vi "Panel.vi"(11 "VerticalSliderControlEditorPanel in":refnum<class "VerticalSliderControlEditorPanel.lvclass">) -> ()   [LabVIEW 2020, in "VolatusGUIControls.lvlib" / "VerticalSliderControlEditorPanel.lvclass"]
uses:
  VerticalSliderControlEditorPanel.lvclass
  C:/dev/lv20CE/relink/volatus-gui-controls/VolatusGUIEditorCore/ElementEditorPanel/ElementEditorPanel.lvclass
  C:/dev/lv20CE/relink/lv-oopanel/OOPanel/Panel/Panel.lvclass
  VolatusGUIEditorCore/Fill Style.ctl
  lv-oopanel/OOPanel/Panel/Basic UI State.ctl
  lv-autocomplete/AutoComplete/AutoComplete/AutoComplete.lvclass/AutoComplete.ctl
  VerticalSliderControlEditorPanel.lvclass/VerticalSliderControlEditorPanel.ctl
  VolatusGUIEditorCore/Slider Props.ctl
  lv-autocomplete/AutoComplete/Launch Autocomplete Handler.vi
  lv-autocomplete/AutoComplete/AutoComplete/AutoComplete.lvclass
  lv-oopanel/OOPanel/Panel/Panel.lvclass
  lv-oopanel/OOPanel/OOPanel.lvlib
  VolatusGUIEditorCore/ElementEditorPanel/ElementEditorPanel.lvclass
  VolatusGUIEditorCore/VolatusGUIEditorCore.lvlib
panel:
  in  "Inhibit":string caption="Channel"
  in  "Max":dbl
  in  "Min":dbl
  in  "Slider Color":u32(colorbox) caption="Slider"
  in  "Fill":T1
  in  "Height":u16
  in  "BG Color":u32(colorbox) caption="BG"
  in  "Fill Color":u32(colorbox) caption="Fill"
  in  "Top":i32
  in  "Left":i32
  in  "Width":u16
  in  "Label Text Color":u32(colorbox) caption="Color"
  in  "Label Visible":bool caption="Visible"
  in  "Label":string
  in  "Channel":string
  # "Label"
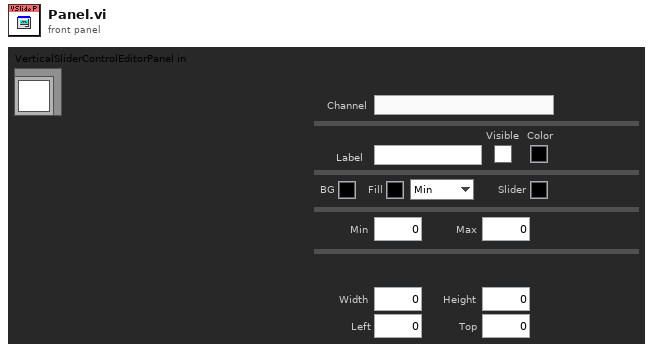
[diagram p1: front panel]
types:
  T1 = typedef "VolatusGUIEditorCore.lvlib/Fill Style.ctl" = enum16{"Min", "Max", "None"}
  T2 = typedef "OOPanel.lvlib/Panel.lvclass/Basic UI State.ctl" = enum16{"Init", "Run", "Close"}
  T3 = typedef "VolatusGUIEditorCore.lvlib/Slider Props.ctl" = cluster{"Fill Color":u32, "BG Color":u32, "Slider Color":u32, "Fill Style":T1, "Min":dbl, "Max":dbl}
  T4 = typedef "VolatusGUIEditorCore.lvlib/ElementEditorPanel.lvclass/Incoming Events.ctl" = cluster{"Update Control":refnum<user-event>}
  T5 = typedef "OOPanel.lvlib/Panel.lvclass/Panel Events.ctl" = cluster{"Visbility":refnum<user-event>, "Close":refnum<user-event>}
  T6 = typedef "VolatusGUIControls.lvlib/VerticalSliderControlEditorPanel.lvclass/Props.ctl" = cluster{"JSON":T7, "Label":T8, "Position":T9, "Width":u16, "Height":u16, "Slider":T3}
  T7 = typedef "VolatusGUIControls.lvlib/VerticalSliderControlEditorPanel.lvclass/JSON Props.ctl" = cluster{"Channel":string, "Inhibit":string}
  T8 = typedef "VolatusGUIEditorCore.lvlib/Label Props.ctl" = cluster{"Text":string, "Text Color":u32, "Visible":bool}
  T9 = typedef "VolatusGUIEditorCore.lvlib/Position Props.ctl" = cluster{"Left":i32, "Top":i32}
  T10 = typedef "OOPanel.lvlib/Visibility State.ctl" = enum16{"Idle", "Closed", "Hidden", "Visible", "Subpanel", "Hidden Subpanel"}
  T11 = cluster{"Label":string, "Label Text Color":u32, "Label Visible":bool}
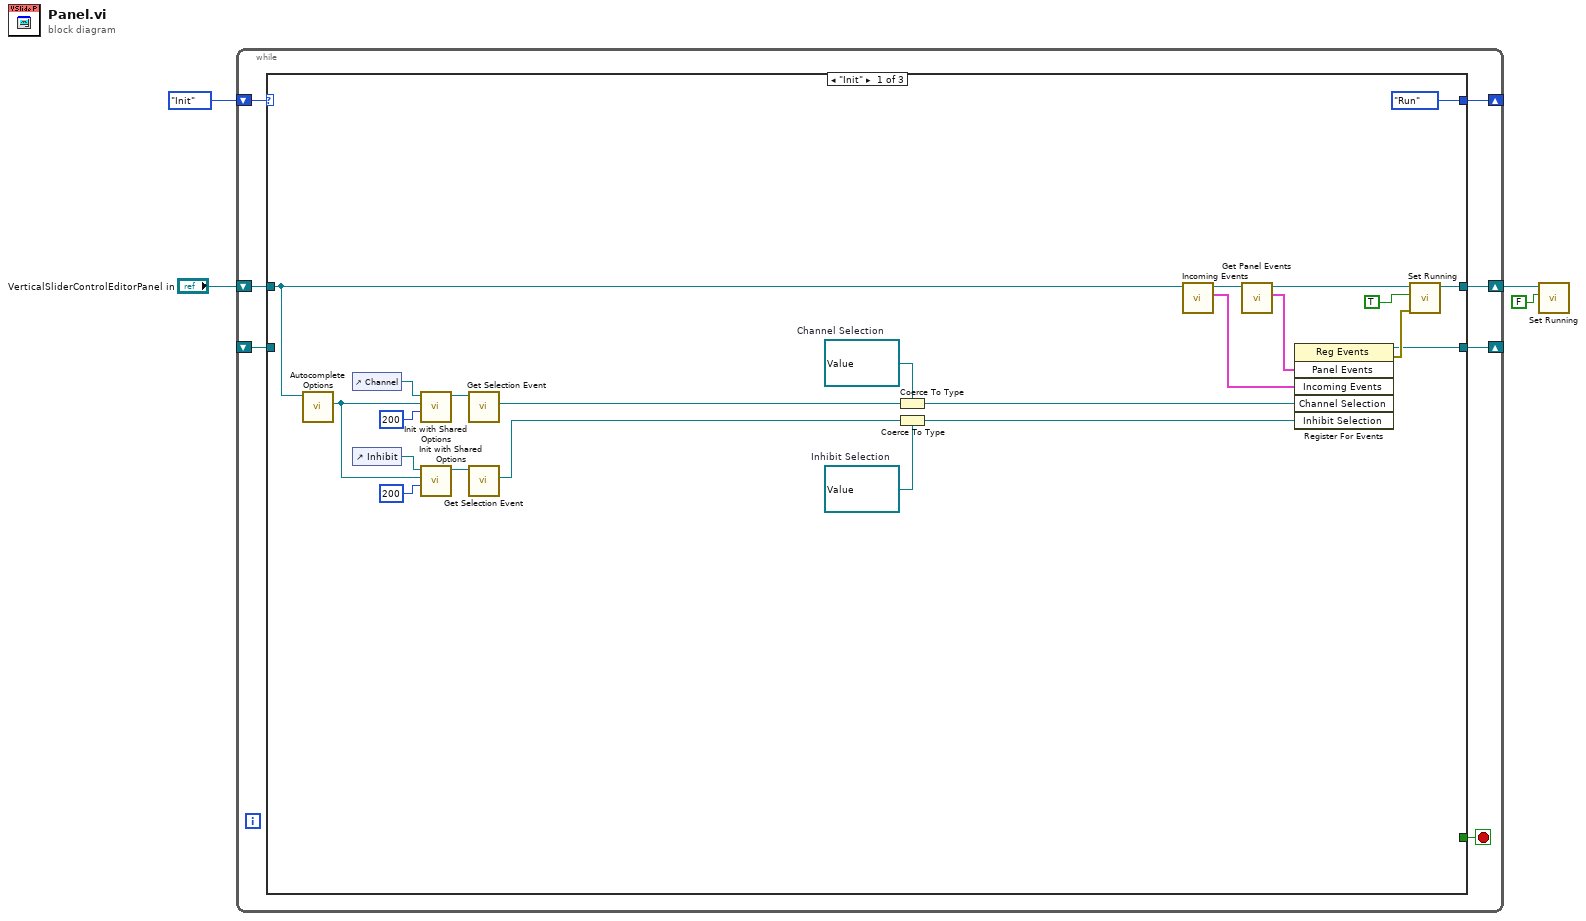
[diagram p0: block diagram]
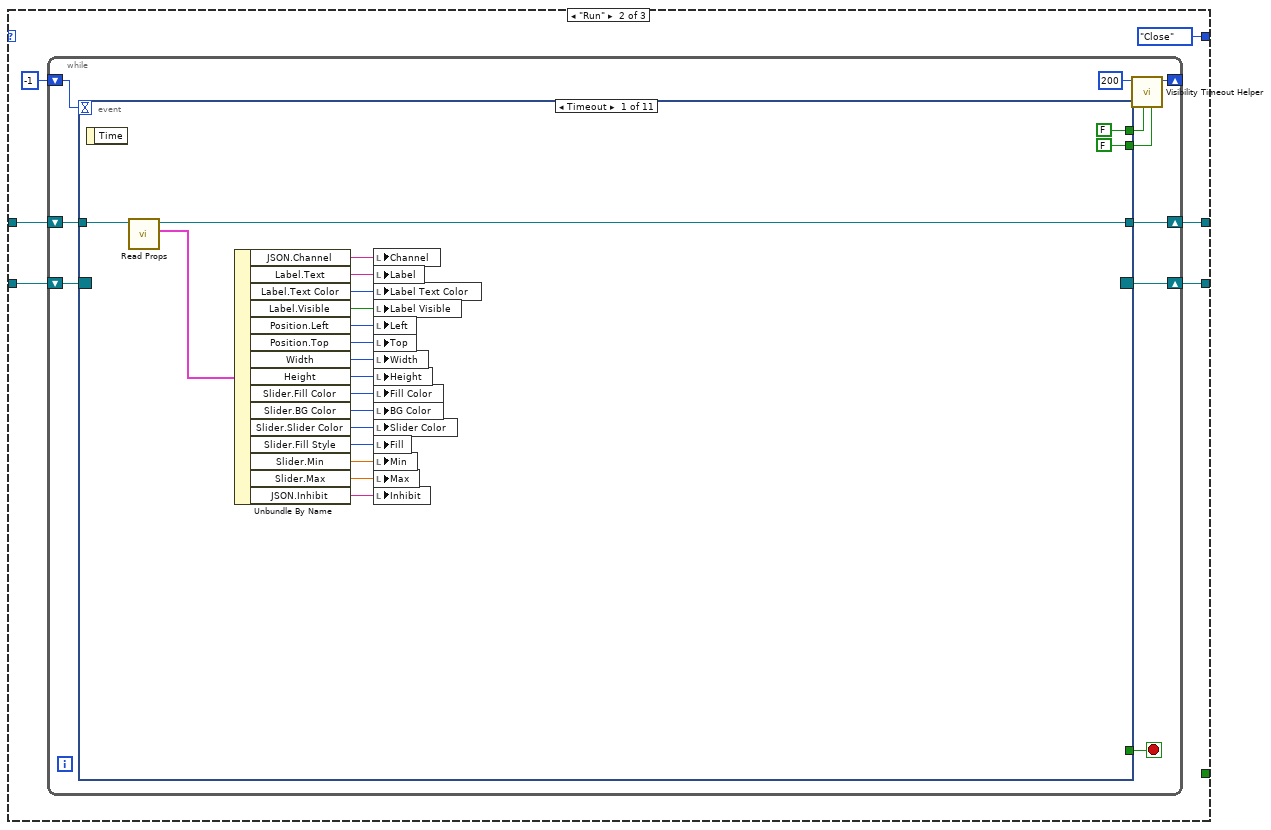
[diagram p2: hidden frame]
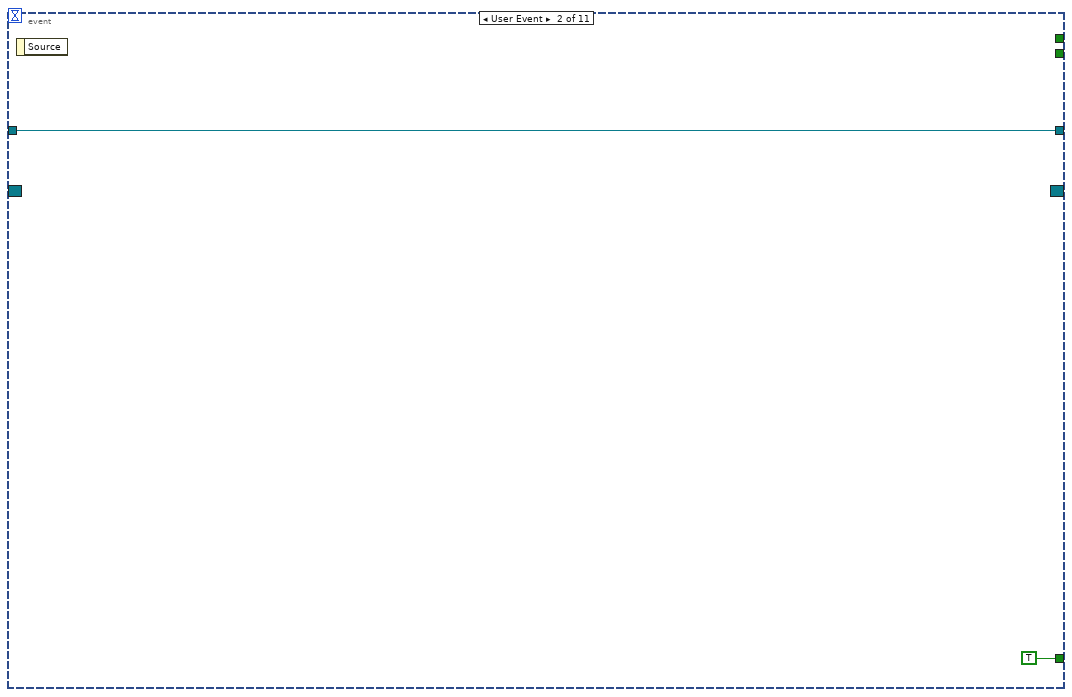
[diagram p3: hidden frame]
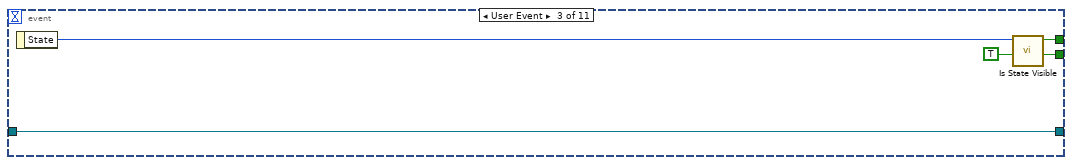
[diagram p4: hidden frame]
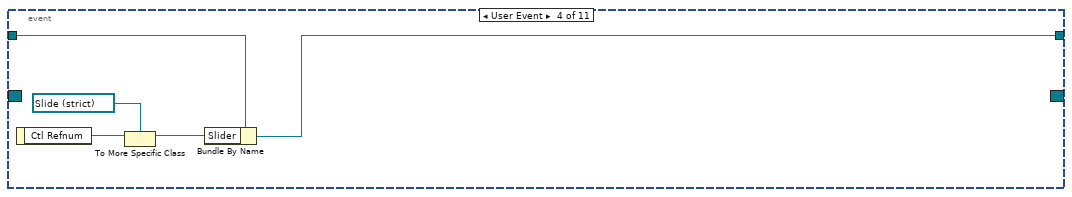
[diagram p5: hidden frame]
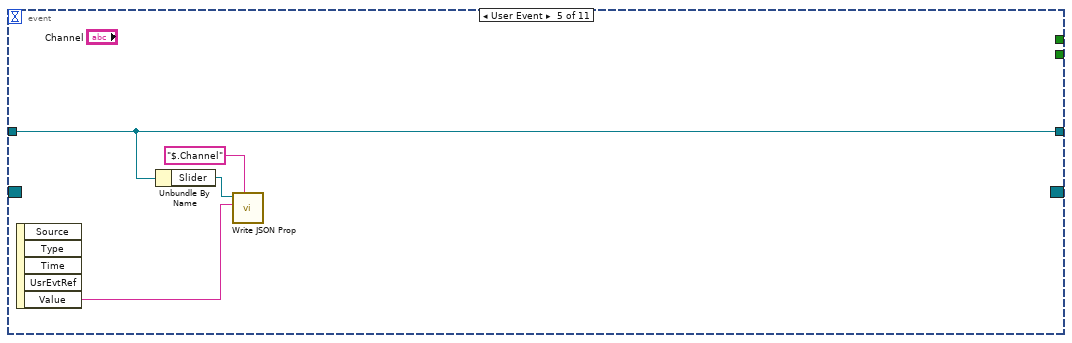
[diagram p6: hidden frame]
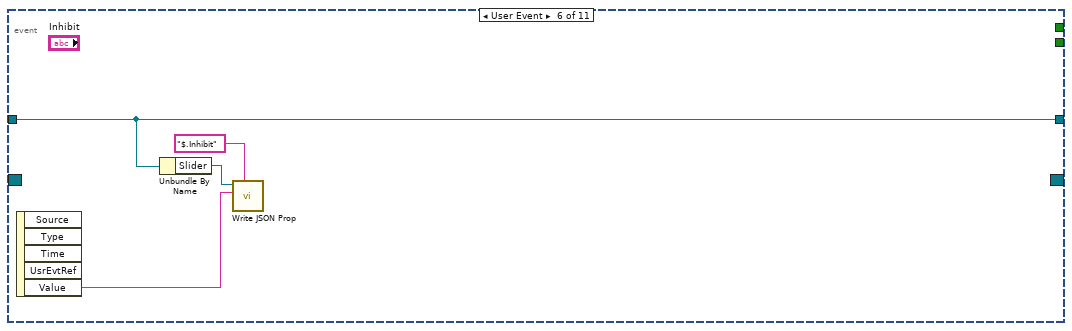
[diagram p7: hidden frame]
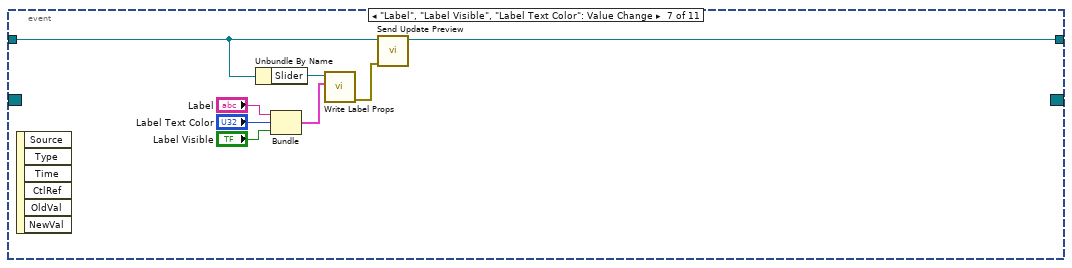
[diagram p8: hidden frame]
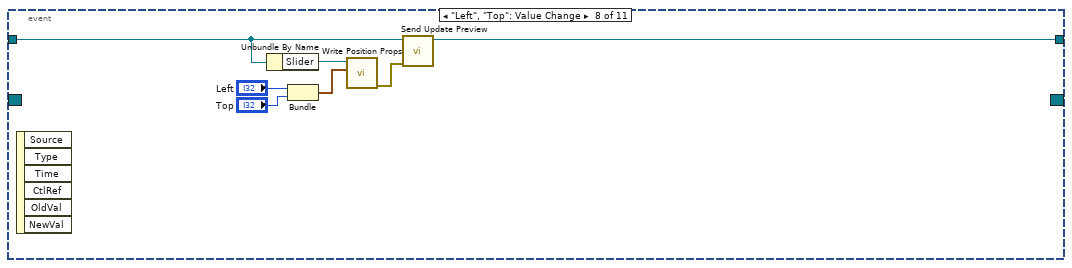
[diagram p9: hidden frame]
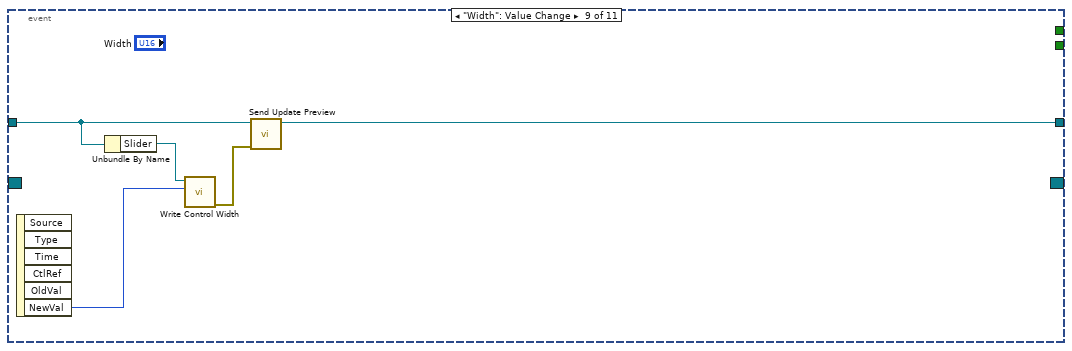
[diagram p10: hidden frame]
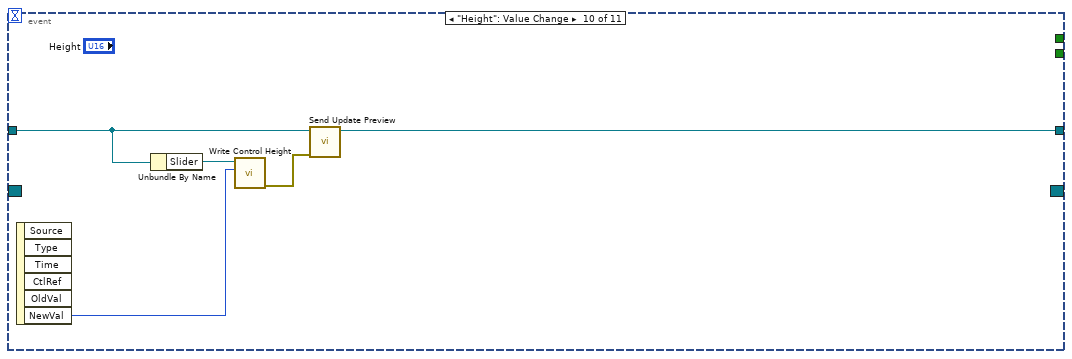
[diagram p11: hidden frame]
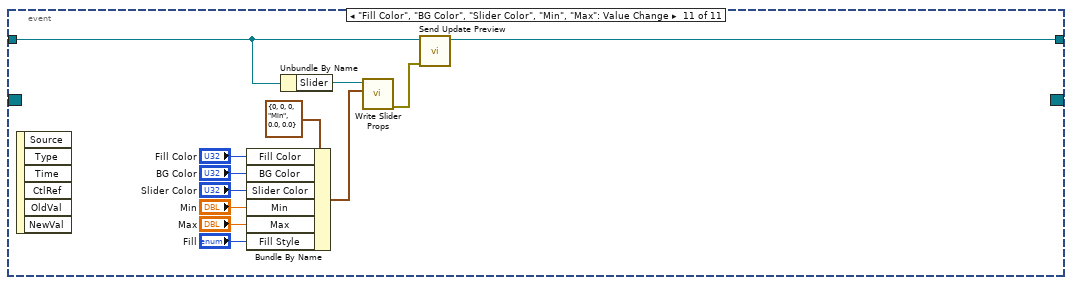
[diagram p12: hidden frame]
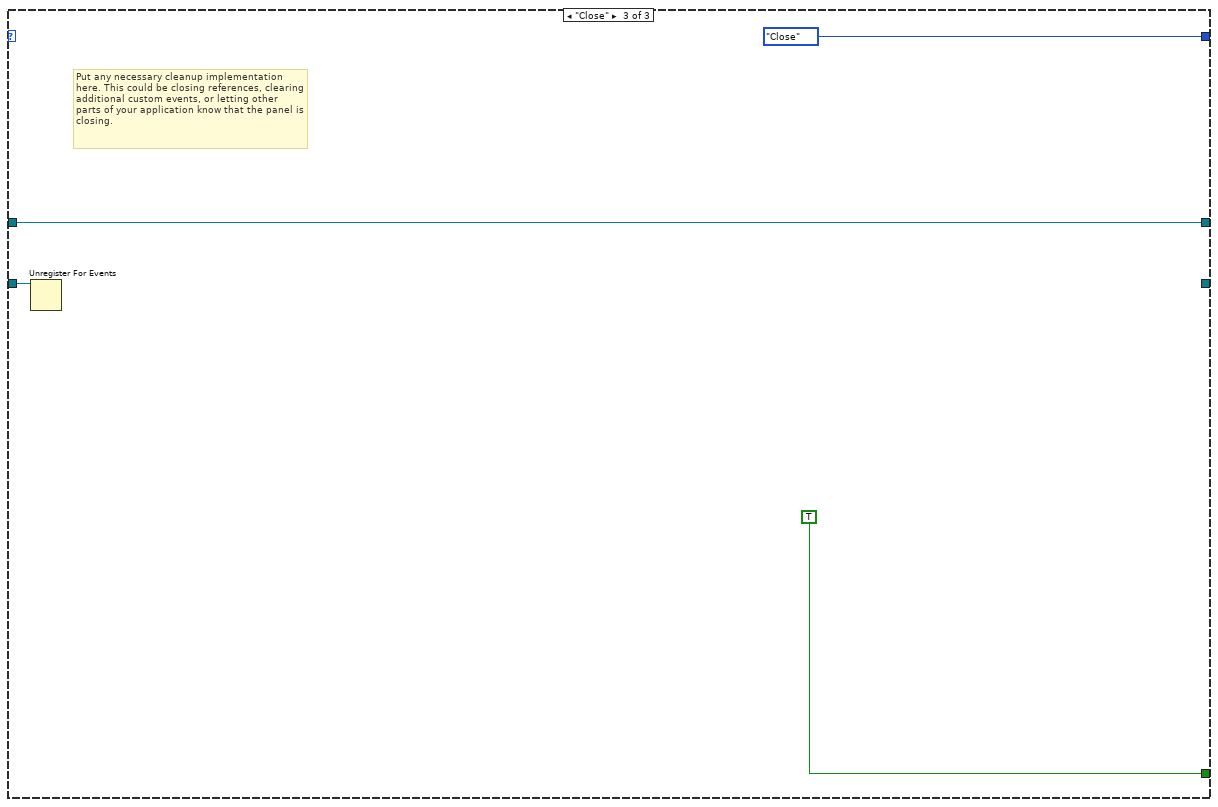
[diagram p13: hidden frame]
diagram:
  n1 = while {
    shift-right: [w10] -> _
    shift-left: _ -> [w11]
    shift-right: [w8] -> _
    shift-left: Basic_UI_State."Init" ("Basic UI State") -> [w9]
    shift-right: [w6] -> w4
    shift-left: "VerticalSliderControlEditorPanel in" -> [w5]
    stop <- w7 stop-if-true
    n2 = case shown="\"Init\"" w9 {
      tunnel: w11 -> [_ w40 w128]
      tunnel: [w31 w38 _] -> w10
      tunnel: [Basic_UI_State."Run" ("Basic UI State") Basic_UI_State."Close" ("Basic UI State") Basic_UI_State."Close" ("Basic UI State")] -> w8
      tunnel: [_ _ TRUE] -> w7
      tunnel: [w30 w35 w127] -> w6
      tunnel: w5 -> [w23 w36 w127]
      frame "Init" {
        w13 = refnum<user-event> refnum  # Inhibit Selection
        w15 = refnum<user-event> refnum  # Channel Selection
        n3 = call "Autocomplete Options.vi"("ElementEditorPanel in"=w23) -> ("Autocomplete Options"=w19:refnum<class "Shared Options.lvclass">)  [unwired: 10 in]
        n4 = control-ref of="Channel"() -> (w22:refnum<vi>)
        n5 = control-ref of="Inhibit"() -> (w17:refnum<vi>)
        n6 = call "Init with Shared Options.vi"("Height (200)"=i16 200, "Shared Options"=w19, "Str Refnum"=w22) -> ("AutoComplete out"=w24:refnum<class "AutoComplete.lvclass">)  [unwired: 7 in, 1 out]
        n7 = call "Init with Shared Options.vi"("Height (200)"=i16 200, "Shared Options"=w19, "Str Refnum"=w17) -> ("AutoComplete out"=w18:refnum<class "AutoComplete.lvclass">)  [unwired: 7 in, 1 out]
        n8 = call "Get Selection Event.vi"("AutoComplete in"=w24) -> ("Selection Event"=w21:refnum<user-event>)  [unwired: 9 in, 1 out]
        n9 = call "Get Selection Event.vi"("AutoComplete in"=w18) -> ("Selection Event"=w12:refnum<user-event>)  [unwired: 9 in, 1 out]
        n10 = Coerce To Type(0:w21, 1:w15) -> (2:w16:refnum<user-event>)
        n11 = Coerce To Type(0:w12, 1:w13) -> (2:w14:refnum<user-event>)
        n12 = call "Incoming Events.vi"("ElementEditorPanel in"=w23) -> ("Incoming Events"=w26:T4, "ElementEditorPanel out"=w27:refnum<class "VerticalSliderControlEditorPanel.lvclass">)  [unwired: 9 in]
        n13 = call "Get Panel Events.vi"("Panel in"=w27) -> ("Panel Events"=w28:T5, "Panel out"=w29:refnum<class "VerticalSliderControlEditorPanel.lvclass">)  [unwired: 8 in, 1 out]
        n14 = register-events(w28, w26, w16, w14) -> (reference out=w31:refnum<event-registration>, error out=w33:errorcluster)  [unwired: 2 in]
        n15 = call "Set Running.vi"("error in (no error)"=w33, "Running"=TRUE, "Panel in"=w29) -> ("Panel out"=w30:refnum<class "VerticalSliderControlEditorPanel.lvclass">)  [unwired: 7 in, 1 out]
      }
      frame "Run" {
        n16 = while {
          shift-right: [w46] -> w38
          shift-left: w40 -> [w47]
          shift-right: [w49] -> _
          shift-left: -1 ("Timeout") -> [w48]
          shift-right: [w41] -> w35
          shift-left: w36 -> [w42]
          stop <- w43 stop-if-true
          n17 = event shown="[0] Timeout" {
            selector: w47 -> [_ _ _ _ _ _ _ _ _ _ _]
            dyn-events: [_ _ _ _ _ _ _ _ _ _ _] -> w46
            timeout: w48 -> [_ _ _ _ _ _ _ _ _ _ _]
            tunnel: [FALSE _ w75 _ _ _ _ _ _ _ _] -> w45
            tunnel: [FALSE _ TRUE _ _ _ _ _ _ _ _] -> w44
            tunnel: [_ TRUE _ _ _ _ _ _ _ _ _] -> w43
            tunnel: w42 -> [w67 w71 w73 w81 w83 w87 w97 w102 w109 w114 w119]
            tunnel: [w68 w71 w73 w78 w83 w87 w91 w99 w106 w111 w116] -> w41
            event Timeout {
              n18 = event-data() -> ()  [unwired: 1 in, 1 out]
              n19 = call "Read Props.vi"("VerticalSliderControlEditorPanel in"=w67) -> ("Props"=w66:T6, "VerticalSliderControlEditorPanel out"=w68:refnum<class "VerticalSliderControlEditorPanel.lvclass">)  [unwired: 8 in, 1 out]
              n20 = Unbundle By Name(w66) -> ("JSON.Channel"=w65:string, "Label.Text"=w63:string, "Label.Text Color"=w62:u32, "Label.Visible"=w61:bool, "Position.Left"=w60:i32, "Position.Top"=w59:i32, "Width"=w58:u16, "Height"=w57:u16, "Slider.Fill Color"=w56:u32, "Slider.BG Color"=w55:u32, "Slider.Slider Color"=w54:u32, "Slider.Fill Style"=w53:T1, "Slider.Min"=w52:dbl, "Slider.Max"=w64:dbl, "JSON.Inhibit"=w51:string)
              n21 = local write "Channel"(w65) -> ()
              n22 = local write "Label"(w63) -> ()
              n23 = local write "Label Text Color"(w62) -> ()
              n24 = local write "Label Visible"(w61) -> ()
              n25 = local write "Left"(w60) -> ()
              n26 = local write "Top"(w59) -> ()
              n27 = local write "Width"(w58) -> ()
              n28 = local write "Height"(w57) -> ()
              n29 = local write "Fill Color"(w56) -> ()
              n30 = local write "BG Color"(w55) -> ()
              n31 = local write "Slider Color"(w54) -> ()
              n32 = local write "Fill"(w53) -> ()
              n33 = local write "Min"(w52) -> ()
              n34 = local write "Max"(w64) -> ()
              n35 = local write "Inhibit"(w51) -> ()
            }
            event User Event {
              n36 = event-data() -> ()  [unwired: 1 in, 1 out]
            }
            event User Event {
              n37 = event-data() -> ("State"=w76:T10)  [unwired: 1 in]
              n38 = call "Is State Visible.vi"("Visibility"=w76) -> ("Visible"=w75:bool)  [unwired: 10 in]
            }
            event User Event {
              n39 = event-data() -> ("Ctl Refnum"=w80:refnum<vi>)  [unwired: 1 in]
              n40 = To More Specific Class(target class=refnum<vi> refnum ("Slide"), reference=w80) -> (specific class reference=w77:refnum<vi>)  [unwired: 1 in, 1 out]
              n41 = Bundle By Name(cluster=w81, "Slider"=w77) -> (w78:refnum<class "VerticalSliderControlEditorPanel.lvclass">)
            }
            event User Event {
              n42 = event-data() -> ("Value"=w82:string)  [unwired: 1 in, 4 out]
              n43 = Unbundle By Name(w83) -> ("Slider"=w85:refnum<vi>)
              n44 = call "Write JSON Prop.vi"("JSON Path"="$.Channel" ("$Path or Item Name"), "Value"=w82, "Ctl Refnum in"=w85) -> ()  [unwired: 7 in, 2 out]
            }
            event User Event {
              n45 = event-data() -> ("Value"=w86:string)  [unwired: 1 in, 4 out]
              n46 = Unbundle By Name(w87) -> ("Slider"=w89:refnum<vi>)
              n47 = call "Write JSON Prop.vi"("JSON Path"="$.Inhibit" ("$Path or Item Name"), "Value"=w86, "Ctl Refnum in"=w89) -> ()  [unwired: 7 in, 2 out]
            }
            event "Label", "Label Visible", "Label Text Color": Value Change {
              n48 = event-data() -> ()  [unwired: 1 in, 6 out]
              n49 = Unbundle By Name(w97) -> ("Slider"=w96:refnum<vi>)
              n50 = Bundle("Label"="Label", "Label Text Color"="Label Text Color", "Label Visible"="Label Visible") -> (w92:T11)  [unwired: 1 in]
              n51 = call "Write Label Props.vi"("Label Props"=w92, "Ctl Refnum in"=w96) -> ("error out"=w90:errorcluster)  [unwired: 8 in, 1 out]
              n52 = call "Send Update Preview.vi"("error in (no error)"=w90, "ElementEditorPanel in"=w97) -> ("ElementEditorPanel out"=w91:refnum<class "VerticalSliderControlEditorPanel.lvclass">)  [unwired: 8 in, 1 out]
            }
            event "Left", "Top": Value Change {
              n53 = event-data() -> ()  [unwired: 1 in, 6 out]
              n54 = Unbundle By Name(w102) -> ("Slider"=w101:refnum<vi>)
              n55 = Bundle("Left"="Left", "Top"="Top") -> (w100:cluster{"Left":i32, "Top":i32})  [unwired: 1 in]
              n56 = call "Write Position Props.vi"("Position Props"=w100, "Ctl Refnum in"=w101) -> ("error out"=w98:errorcluster)  [unwired: 8 in, 1 out]
              n57 = call "Send Update Preview.vi"("error in (no error)"=w98, "ElementEditorPanel in"=w102) -> ("ElementEditorPanel out"=w99:refnum<class "VerticalSliderControlEditorPanel.lvclass">)  [unwired: 8 in, 1 out]
            }
            event "Width": Value Change {
              n58 = event-data() -> ("NewVal"=w107:u16)  [unwired: 1 in, 5 out]
              n59 = Unbundle By Name(w109) -> ("Slider"=w108:refnum<vi>)
              n60 = call "Write Control Width.vi"("Width"=w107, "Control in"=w108) -> ("error out"=w105:errorcluster)  [unwired: 8 in, 1 out]
              n61 = call "Send Update Preview.vi"("error in (no error)"=w105, "ElementEditorPanel in"=w109) -> ("ElementEditorPanel out"=w106:refnum<class "VerticalSliderControlEditorPanel.lvclass">)  [unwired: 8 in, 1 out]
            }
            event "Height": Value Change {
              n62 = event-data() -> ("NewVal"=w112:u16)  [unwired: 1 in, 5 out]
              n63 = Unbundle By Name(w114) -> ("Slider"=w113:refnum<vi>)
              n64 = call "Write Control Height.vi"("Height"=w112, "Control in"=w113) -> ("error out"=w110:errorcluster)  [unwired: 8 in, 1 out]
              n65 = call "Send Update Preview.vi"("error in (no error)"=w110, "ElementEditorPanel in"=w114) -> ("ElementEditorPanel out"=w111:refnum<class "VerticalSliderControlEditorPanel.lvclass">)  [unwired: 8 in, 1 out]
            }
            event "Fill Color", "BG Color", "Slider Color", "Min", "Max": Value Change {
              n66 = event-data() -> ()  [unwired: 1 in, 6 out]
              n67 = Bundle By Name(cluster=T3 {"Fill Color"=0, "BG Color"=0, "Slider Color"=0, "Fill Style"=enum."Min", "Min"=0.0, "Max"=0.0} ("Slider Props"), "Fill Color"="Fill Color", "BG Color"="BG Color", "Slider Color"="Slider Color", "Min"="Min", "Max"="Max", "Fill Style"="Fill") -> (w117:T3)
              n68 = Unbundle By Name(w119) -> ("Slider"=w118:refnum<vi>)
              n69 = call "Write Slider Props.vi"("Slider Props"=w117, "Slider in"=w118) -> ("error out"=w115:errorcluster)  [unwired: 8 in, 1 out]
              n70 = call "Send Update Preview.vi"("error in (no error)"=w115, "ElementEditorPanel in"=w119) -> ("ElementEditorPanel out"=w116:refnum<class "VerticalSliderControlEditorPanel.lvclass">)  [unwired: 8 in, 1 out]
            }
          }
          n71 = call "Visibility Timeout Helper.vi"("Update?"=w44, "Use Timeout?"=w45, "Visible Timeout mS"=200) -> ("Timeout"=w49:i32)  [unwired: 8 in]
        }
      }
      frame "Close" {
        # "Put any necessary cleanup implementation here. This could be closing references, clearing additional custom events, or letting other parts of your application know that the panel is closing."
        n72 = Unregister For Events(event registration refnum=w128) -> ()  [unwired: 1 in, 1 out]
      }
    }
  }
  n73 = call "Set Running.vi"("Running"=FALSE, "Panel in"=w4) -> ()  [unwired: 8 in, 2 out]
